vi "sketch_final.vi"() -> ()   [LabVIEW 2021]
uses:
  sketch_state.ctl
panel:
  in  "Reset":bool
  in  "Left":bool
  in  "UP":bool
  in  "Right":bool
  in  "Down":bool
  in  "stop":bool
  out "Map":picture
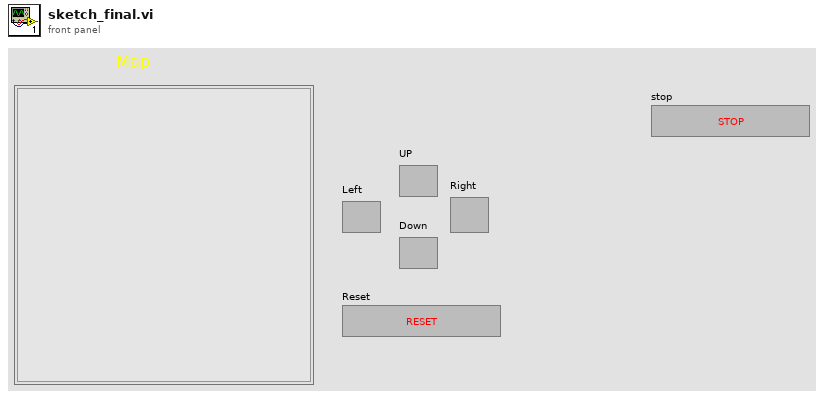
[diagram p1: front panel]
types:
  T1 = typedef "sketch_state.ctl" = enum16{"erase", "wait", "write"}
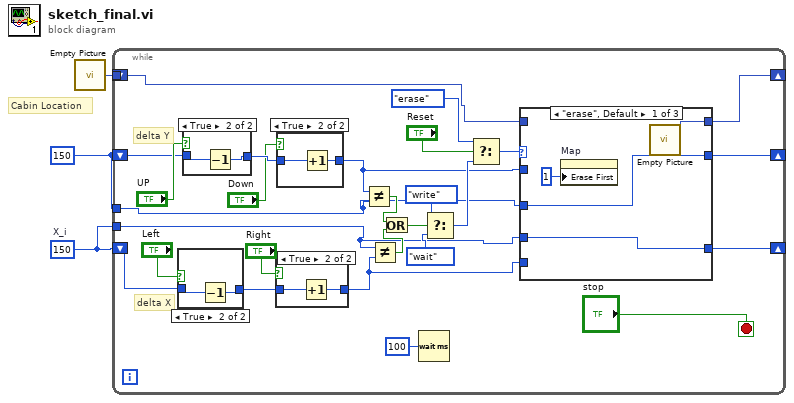
[diagram p0: block diagram]
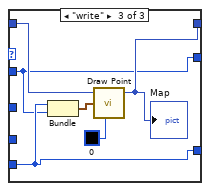
[diagram p3: hidden frame]
diagram:
  w2 = 150 ("Y_i")
  w1 = 150  # X_i
  # "Cabin Location"
  n1 = call "Empty Picture"() -> ("empty picture"=w3:picture)
  n2 = while {
    shift-right: [w6] -> _
    shift-left: w2 -> [w28]
    shift-right: [w5] -> _
    shift-left: w1 -> [w24]
    tunnel: w3 -> [_]
    shift-right: [w20] -> _
    shift-left: _ -> [w21]
    tunnel: w2 -> [w9]
    tunnel: w1 -> [w8]
    stop <- "stop" stop-if-true
    # "delta X"
    # "delta Y"
    n3 = case shown="True" "Left" {
      tunnel: [w50 w52] -> w22
      tunnel: w24 -> [w50 w51]
      frame False {
      }
      frame True {
        n4 = Decrement(x=w51) -> (x-1=w52:i32)
      }
    }
    n5 = case shown="True" "UP" {
      tunnel: [w53 w55] -> w27
      tunnel: w28 -> [w53 w54]
      frame False {
      }
      frame True {
        n6 = Decrement(x=w54) -> (x-1=w55:i32)
      }
    }
    n7 = case shown="True" "Right" {
      tunnel: [w44 w46] -> w7
      tunnel: w22 -> [w44 w45]
      frame False {
      }
      frame True {
        n8 = Increment(x=w45) -> (x+1=w46:i32)
      }
    }
    n9 = case shown="True" "Down" {
      tunnel: [w47 w49] -> w10
      tunnel: w27 -> [w47 w48]
      frame False {
      }
      frame True {
        n10 = Increment(x=w48) -> (x+1=w49:i32)
      }
    }
    n11 = Not Equal?(x=w10, y=w9) -> (x != y?=w17:bool)
    n12 = Not Equal?(x=w8, y=w7) -> (x != y?=w16:bool)
    n13 = Or(x=w17, y=w16) -> (x .or. y?=w15:bool)
    n14 = Wait (ms)(milliseconds to wait=u32 100) -> ()  [unwired: 1 out]
    n15 = Select(t=sketch_state."write", s=w15, f=sketch_state."wait") -> (s? t:f=w12:T1)
    n16 = Select(t=sketch_state."erase", s="Reset", f=w12) -> (s? t:f=w11:T1)
    n17 = case shown="\"erase\", Default" w11 {
      tunnel: w21 -> [_ w37 w41]
      tunnel: [w34 w37 w40] -> w20
      tunnel: w10 -> [_ w36 w38]
      tunnel: w9 -> [w33 _ _]
      tunnel: w8 -> [w32 _ _]
      tunnel: w7 -> [_ w35 w39]
      tunnel: [w33 w36 w38] -> w6
      tunnel: [w32 w35 w39] -> w5
      frame "erase", Default {
        n18 = property on="Map" class="Pict"("Erase First"=u8 1 ("Write Attribute")) -> ()  [unwired: 2 in, 2 out]
        n19 = call "Empty Picture"() -> ("empty picture"=w34:picture)
      }
      frame "wait" {
      }
      frame "write" {
        n20 = Bundle("X_i"=w39, "Y_i"=w38) -> (w42:cluster{"X_i":i32, "Y_i":i32})  [unwired: 1 in]
        n21 = call <vilib>:"Draw Point.vi"("picture"=w41, "point(x,y)"=w42, "color(black)"=u32 0 ("PEN COLOR")) -> ("new picture"=w40:picture)  [unwired: 6 in]
        "Map" <- w40
      }
    }
  }
